vi "NIP Data.vi"() -> (2 "Data":string[](array[string]))   [LabVIEW 2020]
uses:
  Galobal variable_TI.vi
panel:
  out "error out":errorcluster
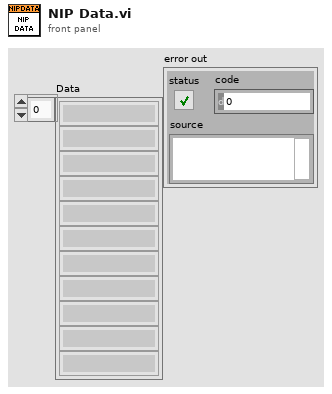
[diagram p1: front panel]
types:
  T1 = cluster{"To-A":timestamp, "From-A":timestamp, "From-B":timestamp, "To-B":timestamp, "From-C 1":timestamp, "To-C 1":timestamp, "From-C 2":timestamp, "To-C 2":timestamp, "Shift":string}
  T2 = cluster{"Stn Name":string, "date":string, "time":string, "Operator id":string, "Shift":string, "Error Code":string, "Fail count":string, "Rework":string, "NA":string, "Tested":string}
  T3 = cluster{"To-A":timestamp, "From-A":timestamp, "From-B":timestamp, "To-B":timestamp, "From-C 1":timestamp, "To-C 1":timestamp, "From-C 2":timestamp, "To-C 2":timestamp}
  T4 = cluster{"No. Fail Coun t":string, "Rework Status Count 0\\1":string, "NA Count Max =3 ":string, "Testesd Count  0/1":string, "Error code":string}
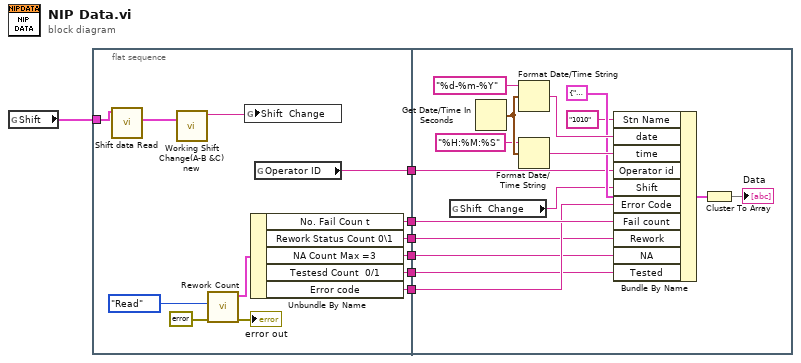
[diagram p0: block diagram]
diagram:
  n1 = global read "Galobal variable_TI.vi" "Shift"() -> (w2:T1)
  n2 = flat-sequence {
    tunnel: [w16] -> w7
    tunnel: [w15] -> w6
    tunnel: [w14] -> w5
    tunnel: [w13] -> w4
    tunnel: [w12] -> w3
    tunnel: w2 -> [w9]
    tunnel: [w8] -> w1
    tunnel: w7 -> [w26]
    tunnel: w6 -> [w25]
    tunnel: w5 -> [w24]
    tunnel: w4 -> [w23]
    tunnel: w3 -> [w22]
    tunnel: w1 -> [w21]
    frame #0 {
      n3 = call "Shift data Read.vi"("input cluster"=w9) -> ("output cluster"=w10:T3)  [unwired: 10 in]
      n4 = call "Working Shift Change(A-B &C) new.vi"("input cluster"=w10) -> ("Shift Change"=w11:string)  [unwired: 10 in]
      n5 = call "Rework Count.vi"("error in"=errorcluster {"status"=FALSE, "code"=0, "source"=""}, "Read /Write"=enum16{"Write", "Read"}."Read") -> ("error out"=→"error out":errorcluster, "data"=w18:T4)  [unwired: 8 in]
      n6 = global write "Galobal variable_TI.vi" "Shift  Change"(w11) -> ()
      n7 = Unbundle By Name(w18) -> ("No. Fail Coun t"=w16:string, "Rework Status Count 0\\1"=w14:string, "NA Count Max =3"=w13:string, "Testesd Count  0/1"=w12:string, "Error code"=w15:string)
      n8 = global read "Galobal variable_TI.vi" "Operator ID"() -> (w8:string)
    }
    frame #1 {
      n9 = global read "Galobal variable_TI.vi" "Shift  Change"() -> (w27:string)
      n10 = Get Date/Time In Seconds() -> (seconds since 1Jan1904=w34:timestamp)
      n11 = Format Date/Time String(time format string (%c)="%d-%m-%Y", seconds (now)=w34) -> (date/time string=w35:string)  [unwired: 1 in]
      n12 = Format Date/Time String(time format string (%c)="%H:%M:%S", seconds (now)=w34) -> (date/time string=w32:string)  [unwired: 1 in]
      n13 = Bundle By Name(cluster=T2 {"Stn Name"="", "date"="", "time"="", "Operator id"="", "Shift"="", "Error Code"="", "Fail count"="", "Rework"="", "NA"="", "Tested"=""} ("Write Data"), "Stn Name"="1010", "date"=w35, "time"=w32, "Operator id"=w21, "Shift"=w27, "Error Code"=w25, "Fail count"=w26, "Rework"=w24, "NA"=w23, "Tested"=w22) -> (w31:T2)
      n14 = Cluster To Array(cluster=w31) -> (array=→"Data":string[])
    }
  }
